vi "Write I2C.vi"(8 "error in (no error)":errorcluster, 10 "LINX I2C":refnum<class "LINX I2C.lvclass">, 11 "LPS25H(B) in":refnum<class "LPS25H(B).lvclass">) -> (0 "error out":errorcluster, 3 "LPS25H(B) out":refnum<class "LPS25H(B).lvclass">)   [LabVIEW 2020, in "LPS25H(B).lvclass"]
uses:
  LPS25H(B).lvclass
  LINX I2C/LINX I2C.lvclass
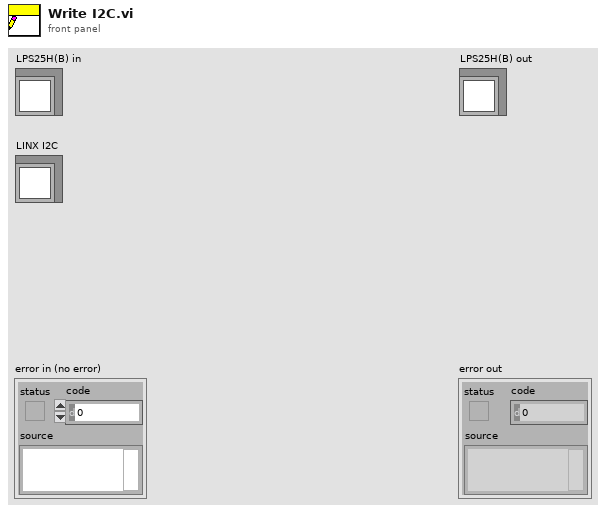
[diagram p1: front panel]
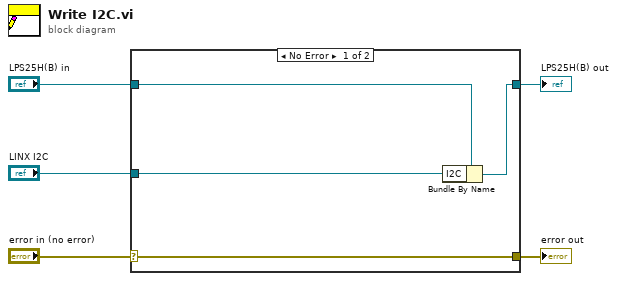
[diagram p0: block diagram]
diagram:
  n1 = case shown="No Error" "error in (no error)" {
    selector: "error in (no error)" -> [w9 w10]
    tunnel: [w9 w10] -> w4
    tunnel: [w7 w11] -> w2
    tunnel: "LPS25H(B) in" -> [w8 w11]
    tunnel: "LINX I2C" -> [w6 _]
    frame No Error {
      n2 = Bundle By Name(cluster=w8, "I2C"=w6) -> (w7:refnum<class "LPS25H(B).lvclass">)
    }
    frame Error {
    }
  }
  "error out" <- w4
  "LPS25H(B) out" <- w2
